vi "PUT In-Place Debug.vi"(0 "In Place Debug Enabled":bool) -> ()   [LabVIEW 2013]
uses:
  src/Functional Globals/Action.ctl
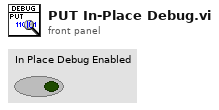
[diagram p1: front panel]
types:
  T1 = typedef "Action.ctl" = enum16{"GET", "PUT", "DELETE"}
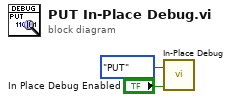
[diagram p0: block diagram]
diagram:
  n1 = call "In-Place Debug.vi"("Input"="In Place Debug Enabled", "Action"=Action."PUT") -> ()  [unwired: 1 in, 1 out]
